vi "change alarm operation.vi"(8 "error in":errorcluster, 9 "boolean op":T1, 10 "alarm name":string, 11 "alarms module configuration in":refnum<class "tag select module configuration.lvclass">=refnum) -> (0 "error out":errorcluster, 3 "alarms module configuration out":refnum<class "tag select module configuration.lvclass">)   [LabVIEW 2013]
doc: "Copyright 2016 National Instruments Corporation\n\nLicensed under the Apache License, Version 2.0 (the \"License\"); you may not use this file except in compliance with the License. You may obtain a copy of the License at http://www.apache.org/licenses/LICENSE-2.0\nUnless required by applicable law or agreed to in writing, software distributed under the License is distributed on an \"AS IS\" BASIS, WITHOUT WARRANTIES OR CONDITIONS OF ANY KIND, either express or implied. See the License for the specific language governing permissions and limitations under the License."
uses:
  <vilib>/tag select/module/configuration/tag select module configuration.lvclass
  boolean operation.ctl
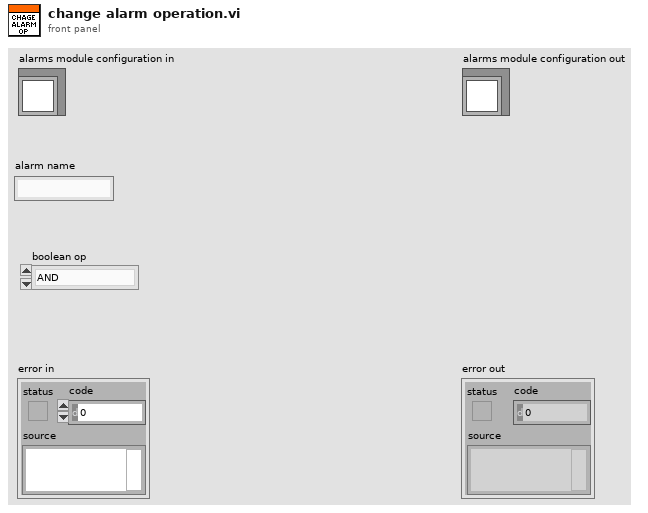
[diagram p1: front panel]
types:
  T1 = typedef "boolean operation.ctl" = enum16{"AND", "OR"}
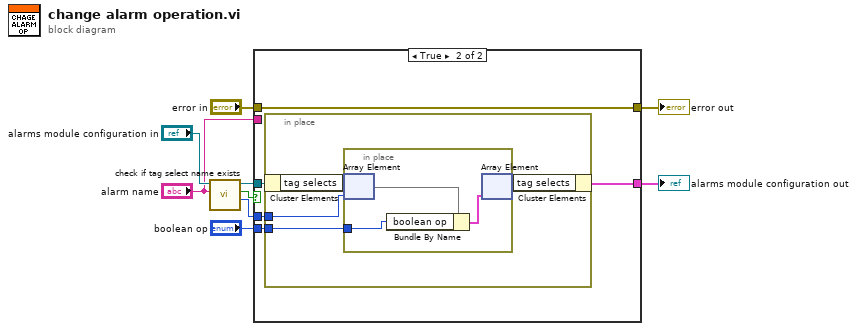
[diagram p0: block diagram]
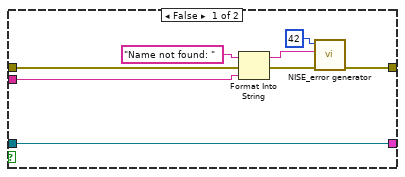
[diagram p2: hidden frame]
diagram:
  n1 = call <vilib>:"check if tag select name exists.vi"("name to locate"="alarm name", "tag select module configuration in"="alarms module configuration in") -> ("index"=w3:i32, "found?"=w6:bool, "tag select module configuration out"=w4:refnum<class "tag select module configuration.lvclass">)  [unwired: 6 in, 1 out]
  n2 = case shown="True" w6 {
    tunnel: [w16 w20] -> w8
    tunnel: "error in" -> [w17 w20]
    tunnel: [w11 w21] -> w5
    tunnel: w4 -> [w11 w22]
    tunnel: w3 -> [_ w19]
    tunnel: "alarm name" -> [w10 _]
    tunnel: "boolean op" -> [_ w18]
    frame False {
      n3 = Format Into String(initial string="Name not found: " ("append error message"), error in=w17, w10) -> (resulting string=w12:string, error out=w14:errorcluster)  [unwired: 1 in]
      n4 = call <vilib>:"NISE_error generator.vi"("error in"=w14, "append error message"=w12, "error code (0)"=42) -> ("error out"=w16:errorcluster)  [unwired: 6 in]
    }
    frame True {
      n5 = in-place {
        in-place-border: w19 -> [w24]
        in-place-border: w18 -> [w23]
        n6 = in-place-cluster #1(w22) -> ("tag selects"=w26)
        n7 = in-place {
          in-place-border: w23 -> [w27]
          n8 = in-place-array #2(w26, w24) -> (w29)
          n9 = Bundle By Name(cluster=w29, "boolean op"=w27) -> (w28:cluster{})
          n10 = in-place-array #2(w28) -> (w25)  [unwired: 1 out]
        }
        n11 = in-place-cluster #1("tag selects"=w25) -> (w21:cluster{})
      }
    }
  }
  "error out" <- w8
  "alarms module configuration out" <- w5
